vi "UTCtime.vi"(11 "UTCtime输入":string) -> (1 "分":i32, 2 "秒":dbl, 3 "时":i32)   [LabVIEW 2018]
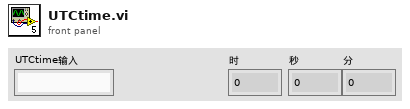
[diagram p1: front panel]
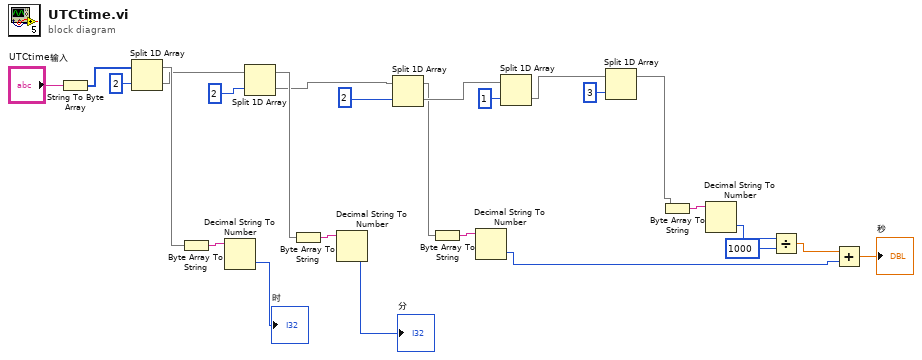
[diagram p0: block diagram]
diagram:
  n1 = String To Byte Array(string="UTCtime输入") -> (unsigned byte array=w25:u8[])
  n2 = Split 1D Array(array=w25, index=2 ("索引")) -> (first subarray=w24:u8[], second subarray=w14:u8[])
  n3 = Byte Array To String(unsigned byte array=w24) -> (string=w18:string)
  n4 = Decimal String To Number(string=w18) -> (number=→"时":i32)  [unwired: 2 in, 1 out]
  n5 = Split 1D Array(array=w14, index=2 ("索引")) -> (first subarray=w13:u8[], second subarray=w12:u8[])
  n6 = Byte Array To String(unsigned byte array=w13) -> (string=w17:string)
  n7 = Decimal String To Number(string=w17) -> (number=→"分":i32)  [unwired: 2 in, 1 out]
  n8 = Split 1D Array(array=w12, index=2 ("索引")) -> (first subarray=w9:u8[], second subarray=w11:u8[])
  n9 = Byte Array To String(unsigned byte array=w9) -> (string=w16:string)
  n10 = Decimal String To Number(string=w16) -> (number=w4:i32)  [unwired: 2 in, 1 out]
  n11 = Split 1D Array(array=w11, index=1 ("索引")) -> (second subarray=w10:u8[])  [unwired: 1 out]
  n12 = Split 1D Array(array=w10, index=3 ("索引")) -> (first subarray=w8:u8[])  [unwired: 1 out]
  n13 = Byte Array To String(unsigned byte array=w8) -> (string=w15:string)
  n14 = Decimal String To Number(string=w15) -> (number=w7:i32)  [unwired: 2 in, 1 out]
  n15 = Divide(x=w7, y=1000) -> (x/y=w5:dbl)
  n16 = Add(x=w5, y=w4) -> (x+y=→"秒":dbl)
